vi "mclb_resize_last.vi"(8 "error in (no error)":errorcluster, 10 "FP.Width":u32, 11 "mclb in":refnum<vi>) -> (0 "error out":errorcluster, 3 "mclb out":refnum<vi>)   [LabVIEW 2017, in "rywindow.lvclass"]
uses:
  rywindow.lvclass
  <vilib>/Utility/miscctls.llb/LVRowAndColumnTypeDef.ctl
panel:
  in  "width 2":i32
  out "width":i32
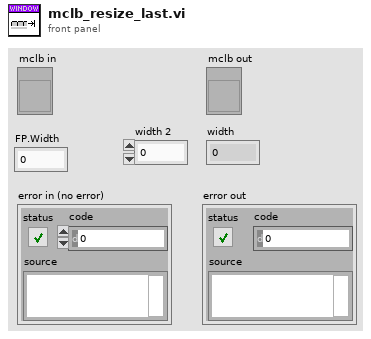
[diagram p1: front panel]
types:
  T1 = typedef "LVRowAndColumnTypeDef.ctl" = cluster{"Row":i32, "Column":i32}
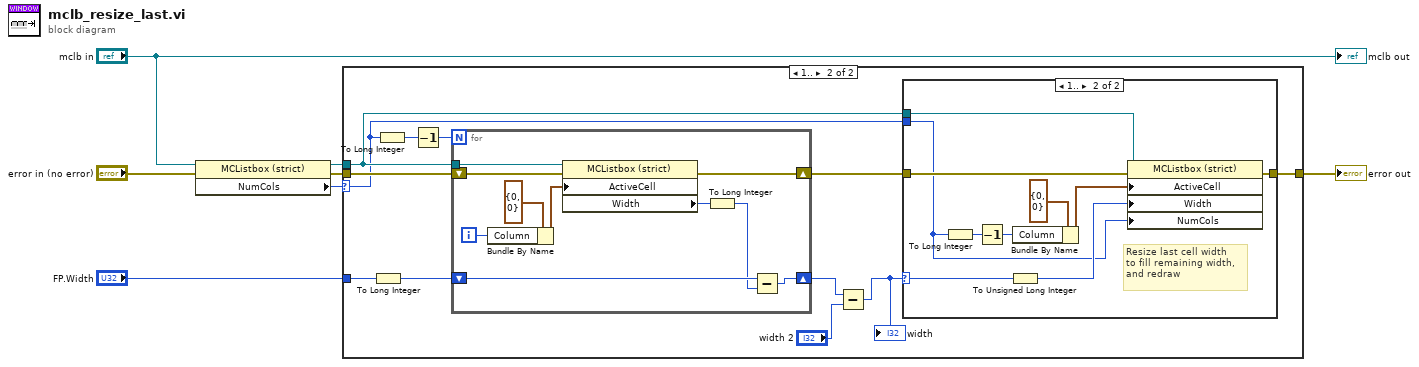
[diagram p0: block diagram]
diagram:
  n1 = property class="MCListbox (strict)"(reference="mclb in", error in="error in (no error)") -> (reference out=w6:refnum<vi>, error out=w5:errorcluster, "NumCols"=w4:u32)
  n2 = case shown="1.." w4 {
    selector: w4 -> [_ w12]
    tunnel: w5 -> [w8 w20]
    tunnel: [w8 w14] -> w2
    tunnel: w6 -> [_ w16]
    tunnel: "FP.Width" -> [_ w19]
    frame 0, Default {
    }
    frame 1.. {
      n3 = To Long Integer(number=w19) -> (32bit integer=w18:i32)
      n4 = To Long Integer(number=w12) -> (32bit integer=w13:i32)
      n5 = Decrement(x=w13) -> (x-1=w15:i32)
      n6 = for {
        N: w15 -> [_]
        tunnel: w16 -> [w38]
        shift-right: [w39] -> w17
        shift-left: w20 -> [w41]
        shift-right: [w33] -> w10
        shift-left: w18 -> [w35]
        i -> [w36]
        n7 = Bundle By Name(cluster=T1 {"Row"=0, "Column"=0} ("Active Cell:Active Cell"), "Column"=w36) -> (w37:T1)
        n8 = property class="MCListbox (strict)"(reference=w38, error in=w41, "ActiveCell"=w37) -> (error out=w39:errorcluster, "Width"=w34:u32)  [unwired: 1 out]
        n9 = To Long Integer(number=w34) -> (32bit integer=w32:i32)
        n10 = Subtract(x=w35, y=w32) -> (x-y=w33:i32)
      }
      n11 = Subtract(x=w10, y="width 2") -> (x-y=w9:i32)
      "width" <- w9
      n12 = case shown="1.." w9 {
        selector: w9 -> [_ w26]
        tunnel: w17 -> [w21 w29]
        tunnel: w16 -> [_ w28]
        tunnel: w12 -> [_ w23]
        tunnel: [w21 w27] -> w14
        frame 0, Default {
        }
        frame 1.. {
          # "Resize last cell width\nto fill remaining width,\nand redraw"
          n13 = To Long Integer(number=w23) -> (32bit integer=w22:i32)
          n14 = Decrement(x=w22) -> (x-1=w24:i32)
          n15 = To Unsigned Long Integer(number=w26) -> (unsigned 32bit integer=w25:u32)
          n16 = Bundle By Name(cluster=T1 {"Row"=0, "Column"=0} ("Active Cell:Active Cell"), "Column"=w24) -> (w31:T1)
          n17 = property class="MCListbox (strict)"(reference=w28, error in=w29, "ActiveCell"=w31, "Width"=w25, "NumCols"=w23) -> (error out=w27:errorcluster)  [unwired: 1 out]
        }
      }
    }
  }
  "error out" <- w2
  "mclb out" <- "mclb in"
